vi "Tag Names.vi"(11 "Process Name":string) -> (3 "Pump Module Tag Names":T1, 4 "All Boolean Tags":string[](array[string]), 5 "All  Numeric Tags":string[](array[string]))   [LabVIEW 2018, in "D-O Module.lvlib" / "D-O Module Engine.lvlib"]
uses:
  D-O Module Engine.lvlib
  D-O Module Tag Names Cluster.ctl
  D-O Module.lvlib
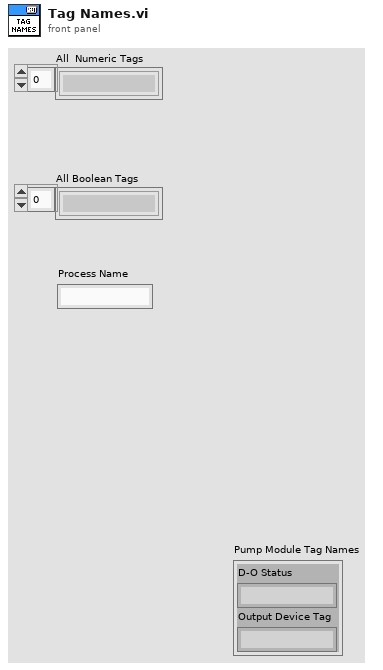
[diagram p1: front panel]
types:
  T1 = typedef "D-O Module.lvlib/D-O Module Tag Names Cluster.ctl" = cluster{"D-O Status":string, "Output Device Tag":string}
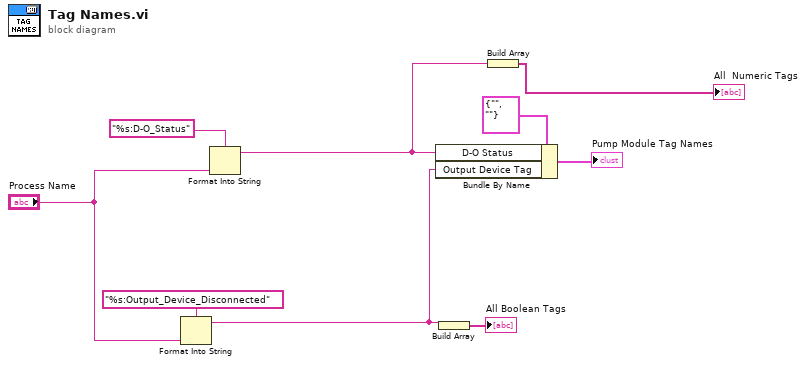
[diagram p0: block diagram]
diagram:
  n1 = Format Into String(format string="%s:Output_Device_Disconnected", "Process Name") -> (resulting string=w8:string)  [unwired: 2 in, 1 out]
  n2 = Format Into String(format string="%s:D-O_Status", "Process Name") -> (resulting string=w2:string)  [unwired: 2 in, 1 out]
  n3 = Bundle By Name(cluster=T1 {"D-O Status"="", "Output Device Tag"=""} ("Feed Module Tag Names"), "D-O Status"=w2, "Output Device Tag"=w8) -> (→"Pump Module Tag Names":T1)
  n4 = Build Array(w8) -> (→"All Boolean Tags":string[])
  n5 = Build Array(w2) -> (→"All  Numeric Tags":string[])
